vi "GetDeviceScanEvent.vi"(8 "错误输入（无错误）":errorcluster, 10 "ArraySize":i32, 11 "返回事件数组":u8[](array[numeric])) -> (0 "错误输出":errorcluster, 3 "返回事件数组":u8[](array[numeric]))   [LabVIEW 2014]
uses:
  ZXUTConfigMgr.dll
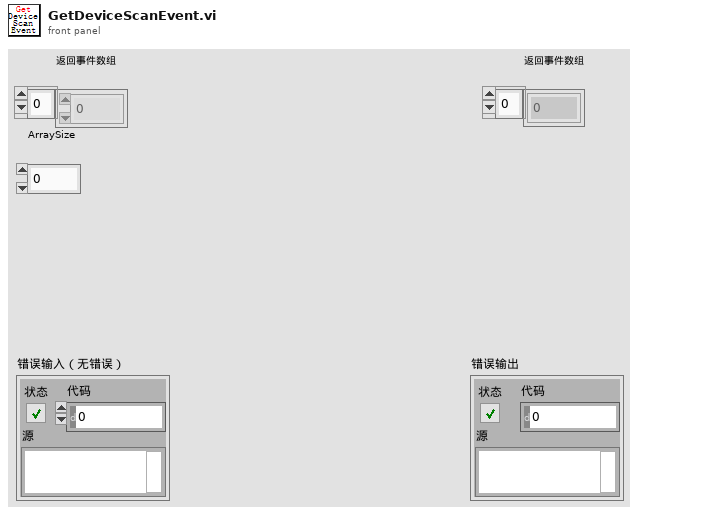
[diagram p1: front panel]
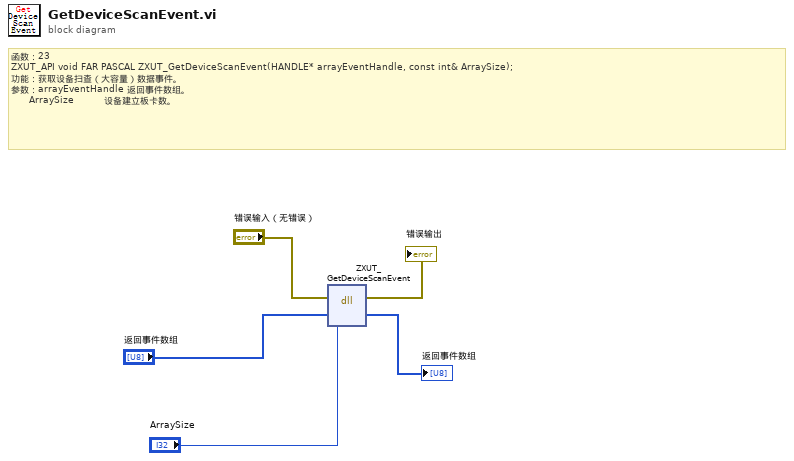
[diagram p0: block diagram]
diagram:
  # "函数：23\nZXUT_API void\tFAR PASCAL ZXUT_GetDeviceScanEvent(HANDLE* arrayEventHandle, const int& ArraySize);\n功能：获取设备扫查（大容量）数据事件。\n参数：arrayEventHandle 返回事件数组。\n      ArraySize          设备建立板卡数。"
  n1 = dll-call lib="PTH2eabs D软件超声实时监测软件ZXUTAppDemo(华南理工V02.00)X86DllZXUTConfigMgr.dll" fn="ZXUT_GetDeviceScanEvent"(error in="错误输入（无错误）", "arrayEventHandle"="返回事件数组", "ArraySize"="ArraySize") -> (error out=→"错误输出":errorcluster, "arrayEventHandle"=→"返回事件数组":u8[])  [unwired: 4 in, 1 out]
